vi "2 XYPointsToDistanceAndAngle.vi"(8 "East 2":dbl, 9 "North 2":dbl, 10 "East 1":dbl, 11 "North 1":dbl) -> (2 "Angle Diff":dbl, 3 "Distance":dbl)   [LabVIEW 2011]
doc: "given two points in cartesian coordinates, this VI outputs the distance between them and the angle from the vertical to the line connecting the two points"
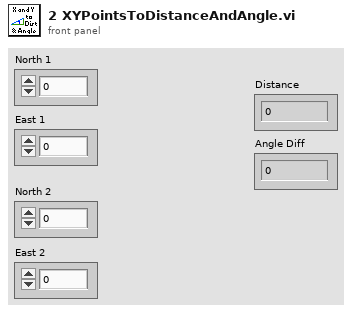
[diagram p1: front panel]
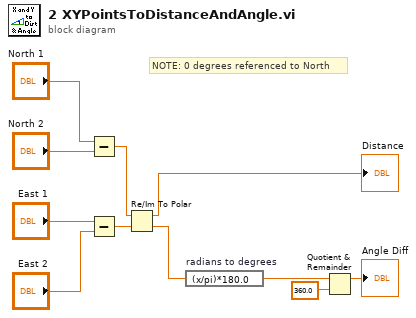
[diagram p0: block diagram]
diagram:
  # "NOTE: 0 degrees referenced to North"
  n1 = Subtract(x="North 1", y="North 2") -> (x-y=w3:dbl)
  n2 = Subtract(x="East 1", y="East 2") -> (x-y=w6:dbl)
  n3 = Re/Im To Polar(2:w6, 3:w3) -> (0:w7:dbl, 1:→"Distance":dbl)
  n4 = expression code="(x/pi)*180.0" "radians to degrees"(w7) -> (w5:dbl)
  n5 = Quotient & Remainder(x=w5, y=360.0) -> (x-y*floor(x/y)=→"Angle Diff":dbl)  [unwired: 1 out]
